vi "Get Free Label Text.vi"(8 "Error In":errorcluster, 10 "Process Bold Characters?":bool, 11 "Free Label Ref":refnum<vi>) -> (0 "Error Out":errorcluster, 2 "Processing Time (ms)":dbl format="%.3f", 3 "VI Description Text":string)   [LabVIEW 2022 SP3]
panel:
  # "Input\nInputs to the VI"
  # "Development\nControls or indicators that are useful for development or testing, but which are not outputs of the VI."
  # "Output\nOutputs of the VI"
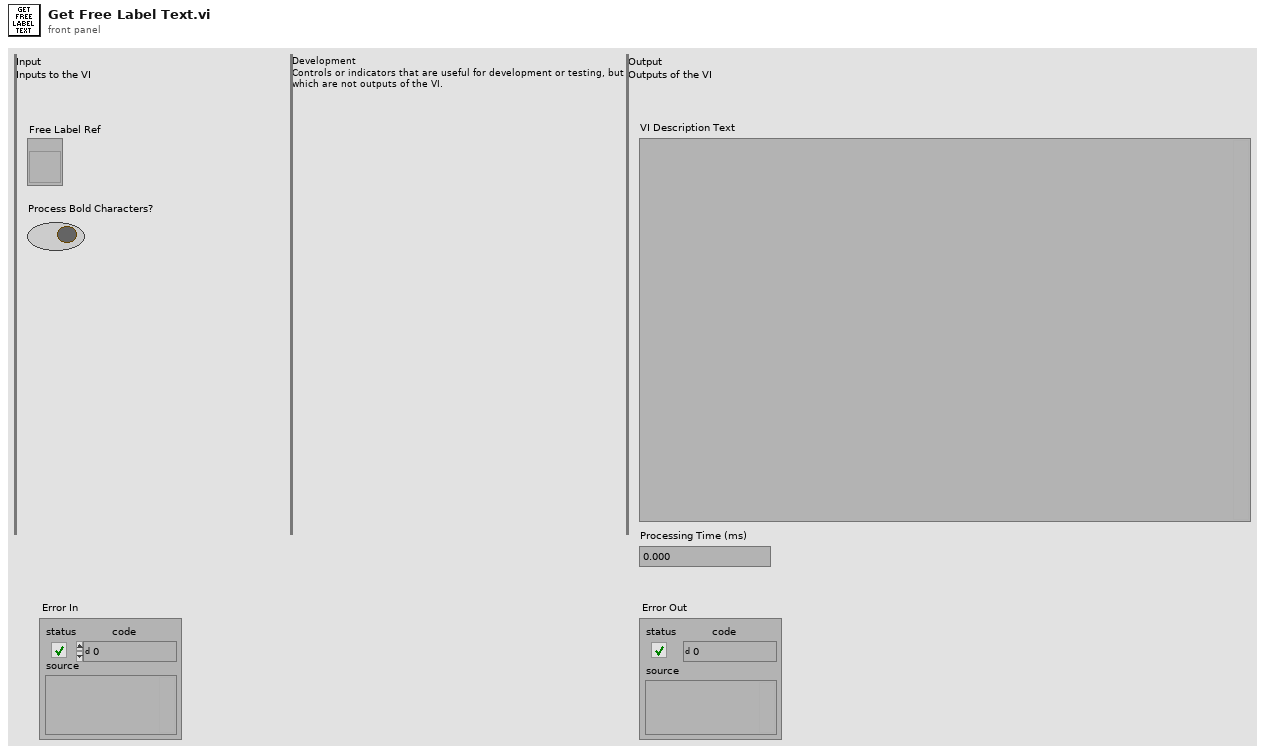
[diagram p1: front panel]
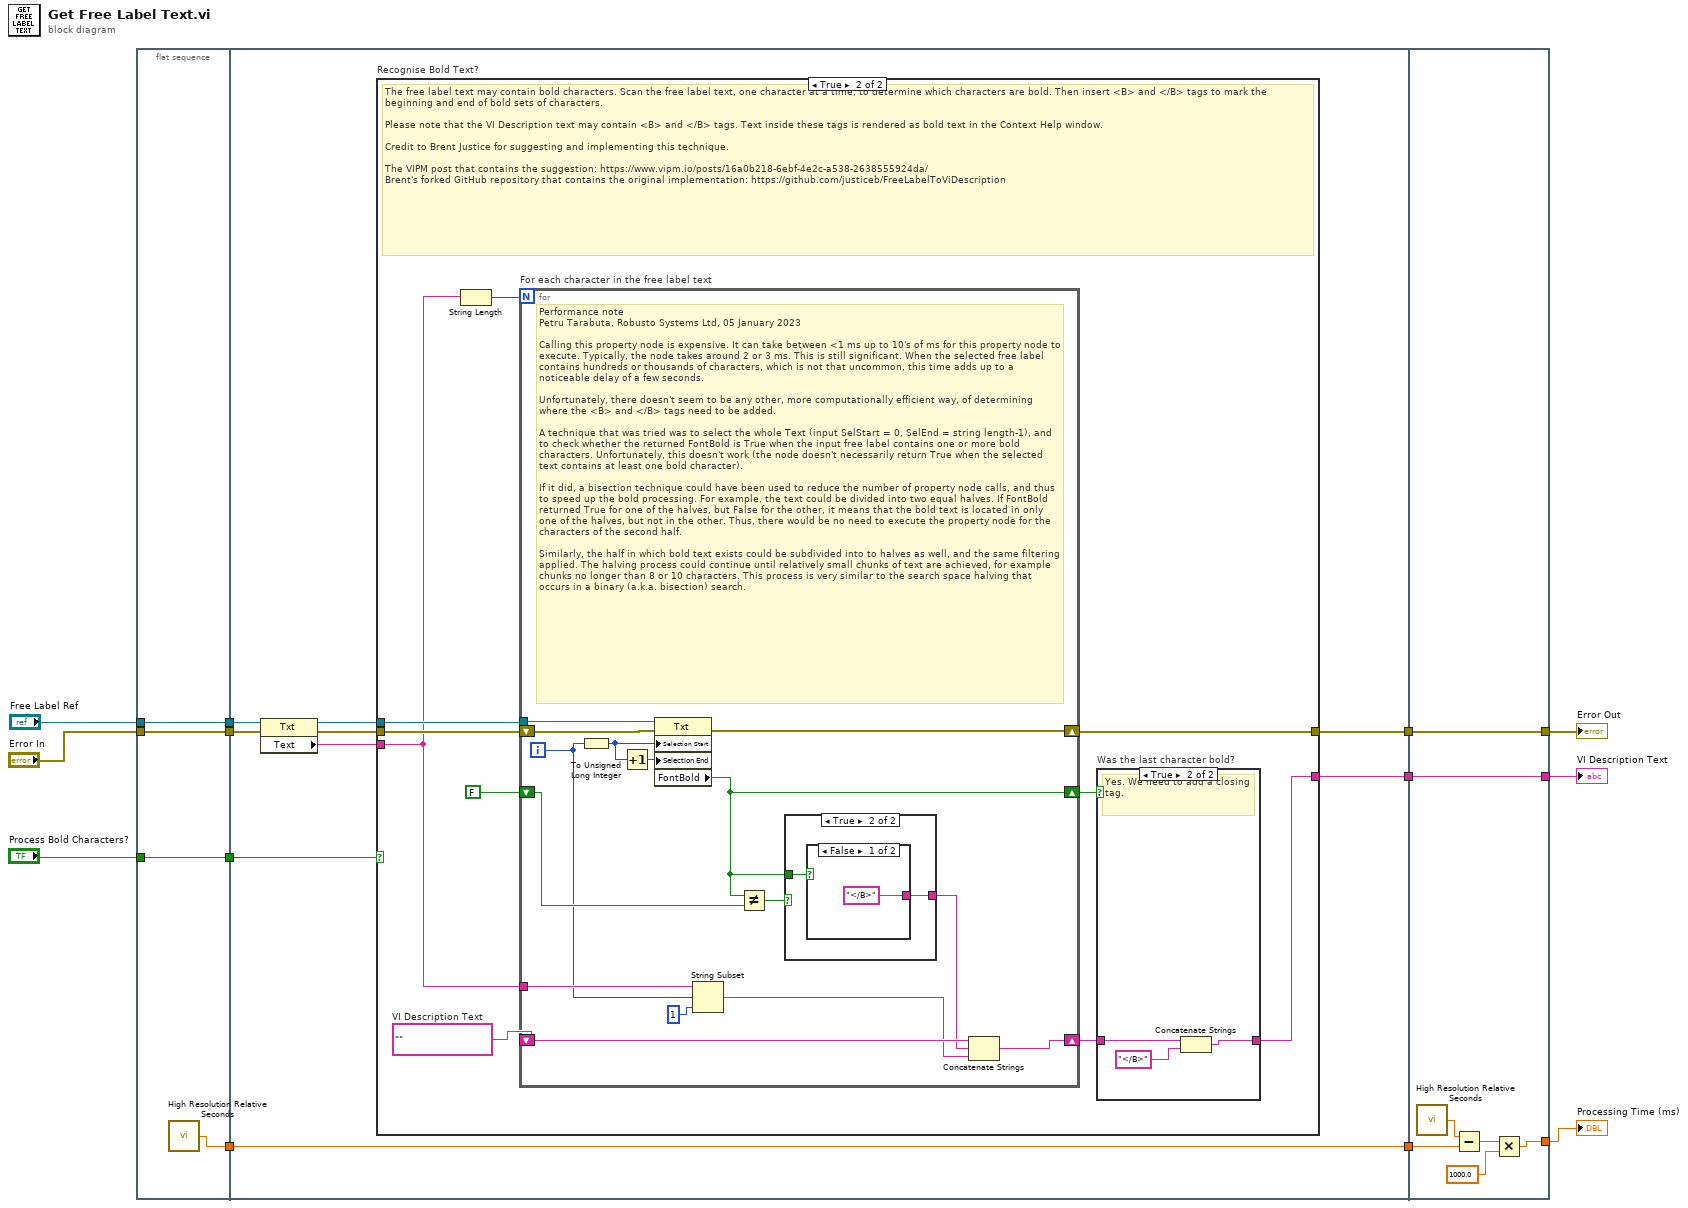
[diagram p0: block diagram]
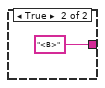
[diagram p4: hidden frame]
diagram:
  n1 = flat-sequence {
    tunnel: "Error In" -> [w16]
    tunnel: "Free Label Ref" -> [w17]
    tunnel: [w17] -> w8
    tunnel: [w16] -> w7
    tunnel: [w15] -> w5
    tunnel: [w14] -> w2
    tunnel: "Process Bold Characters?" -> [w14]
    tunnel: [w25] -> w10
    tunnel: [w24] -> w9
    tunnel: w8 -> [w20]
    tunnel: w7 -> [w26]
    tunnel: [w23] -> w6
    tunnel: w5 -> [w23]
    tunnel: w2 -> [w22]
    tunnel: [w67] -> w11
    tunnel: [w68] -> w12
    tunnel: w10 -> [w68]
    tunnel: w9 -> [w67]
    tunnel: w6 -> [w65]
    tunnel: [w63] -> w4
    frame #0 {
      n2 = call <vilib>:"High Resolution Relative Seconds.vi"() -> ("relative seconds"=w15:dbl)
    }
    frame #1 {
      n3 = property class="Txt"(reference=w20, error in=w26) -> (reference out=w19:refnum<vi>, error out=w21:errorcluster, "Text"=w18:string)
      n4 = case "Recognise Bold Text?" shown="True" w22 {
        tunnel: w19 -> [_ w38]
        tunnel: w21 -> [w28 w34]
        tunnel: [w28 w33] -> w25
        tunnel: [w27 w30] -> w24
        tunnel: w18 -> [w27 w29]
        frame False {
          # "The VI Description text won't contain any <B> or </B> tags."
        }
        frame True {
          w36 = ""  # VI Description Text
          # "The free label text may contain bold characters. Scan the free label text, one character at a time, to determine which characters are bold. Then insert <B> and </B> tags to mark the beginning and end of bold sets of characters.\n\nPlease note that the VI Description text may contain <B> and </B> tags. Text inside these tags is rendered as bold text in the Context Help window.\n\nCredit to Brent Justice for suggesting and implementing this technique.\n\nThe VIPM post that contains the suggestion: https://www.vipm.io/posts/16a0b218-6ebf-4e2c-a538-2638555924da/\nBrent's forked GitHub repository that contains the original implementation: https://github.com/justiceb/FreeLabelToViDescription"
          n5 = String Length(string=w29) -> (length=w37:i32)
          n6 = for "For each character in the free label text" {
            N: w37 -> [_]
            tunnel: w38 -> [w53]
            tunnel: w29 -> [w50]
            shift-right: [w43] -> w31
            shift-left: w36 -> [w46]
            shift-right: [w47] -> w32
            shift-left: FALSE ("Font:Bold") -> [w49]
            shift-right: [w41] -> w33
            shift-left: w34 -> [w42]
            i -> [w40]
            # "Performance note\nPetru Tarabuta, Robusto Systems Ltd, 05 January 2023\n\nCalling this property node is expensive. It can take between <1 ms up to 10's of ms for this property node to execute. Typically, the node takes around 2 or 3 ms. This is still significant. When the selected free label contains hundreds or thousands of characters, which is not that uncommon, this time adds up to a noticeable delay of a few seconds.\n\nUnfortunately, there doesn't seem to be any other, more computationally efficient way, of determining where the <B> and </B> tags need to be added.\n\nA technique that was tried was to select the whole Text (input SelStart = 0, SelEnd = string length-1), and to check whether the returned FontBold is True when the input free label contains one or more bold characters. Unfortunately, this doesn't work (the node doesn't necessarily return True when the selected text contains at least one bold character).\n\nIf it did, a bisection technique could have been used to reduce the number of property node calls, and thus to speed up the bold processing. For example, the text could be divided into two equal halves. If FontBold returned True for one of the halves, but False for the other, it means that the bold text is located in only one of the halves, but not in the other. Thus, there would be no need to execute the property node for the characters of the second half.\n\nSimilarly, the half in which bold text exists could be subdivided into to halves as well, and the same filtering applied. The halving process could continue until relatively small chunks of text are achieved, for example chunks no longer than 8 or 10 characters. This process is very similar to the search space halving that occurs in a binary (a.k.a. bisection) search."
            n7 = To Unsigned Long Integer(number=w40) -> (unsigned 32bit integer=w39:u32)
            n8 = Increment(x=w39) -> (x+1=w52:u32)
            n9 = property class="Txt"(reference=w53, error in=w42, "Selection Start"=w39, "Selection End"=w52) -> (error out=w41:errorcluster, "FontBold"=w47:bool)  [unwired: 1 out]
            n10 = String Subset(string=w50, offset (0)=w40, length (rest)=1 ("length (rest)")) -> (substring=w44:string)
            n11 = Not Equal?(x=w47, y=w49) -> (x != y?=w48:bool)
            n12 = case shown="True" w48 {
              tunnel: w47 -> [_ w55]
              tunnel: [_ w54] -> w45
              frame False {
              }
              frame True {
                n13 = case shown="False" w55 {
                  tunnel: ["</B>" "<B>"] -> w54
                  frame False {
                  }
                  frame True {
                  }
                }
              }
            }
            n14 = Concatenate Strings(w46, w45, w44) -> (w43:string)
          }
          n15 = case "Was the last character bold?" shown="True" w32 {
            tunnel: w31 -> [w58 w61]
            tunnel: [w58 w59] -> w30
            frame False {
              # "No. No need to add any more tags. Do nothing."
            }
            frame True {
              # "Yes. We need to add a closing tag."
              n16 = Concatenate Strings(w61, "</B>") -> (w59:string)
            }
          }
        }
      }
    }
    frame #2 {
      n17 = call <vilib>:"High Resolution Relative Seconds.vi"() -> ("relative seconds"=w66:dbl)
      n18 = Subtract(x=w66, y=w65) -> (x-y=w64:dbl)
      n19 = Multiply(x=w64, y=1000.0) -> (x*y=w63:dbl)
    }
  }
  "VI Description Text" <- w11
  "Error Out" <- w12
  "Processing Time (ms)" <- w4
